vi "2. Simple State Machine Traffic Light.vi"() -> ()   [LabVIEW 2018]
panel:
  in  "stop":bool
  out "Green":bool
  out "Yellow":bool
  out "Red":bool
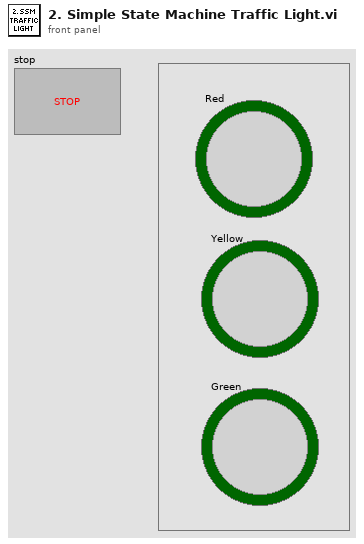
[diagram p1: front panel]
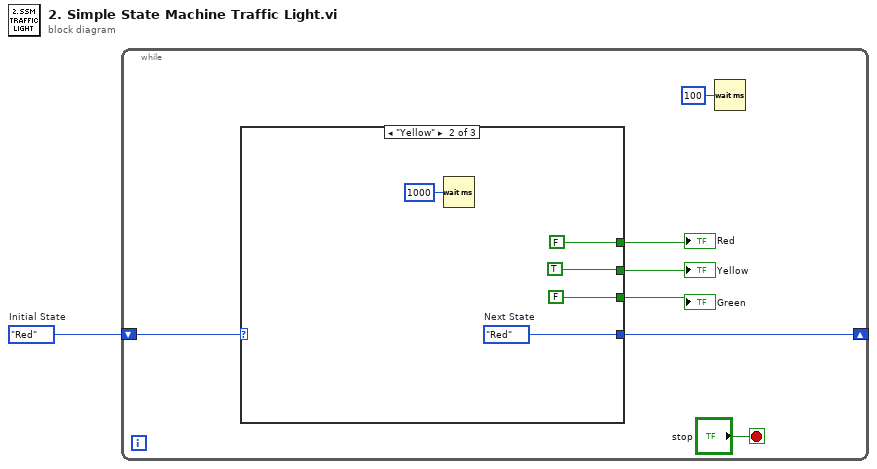
[diagram p0: block diagram]
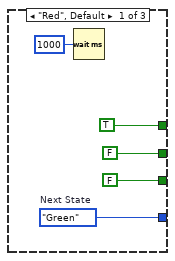
[diagram p2: hidden frame]
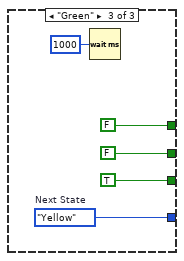
[diagram p3: hidden frame]
diagram:
  w1 = enum16{"Red", "Yellow", "Green"}."Red"  # Initial State
  n1 = while {
    shift-right: [w7] -> _
    shift-left: w1 -> [w8]
    stop <- "stop" stop-if-true
    n2 = case shown="\"Yellow\"" w8 {
      tunnel: [TRUE FALSE FALSE] -> w2
      tunnel: [w12 w17 w22] -> w7
      tunnel: [FALSE TRUE FALSE] -> w4
      tunnel: [FALSE FALSE TRUE] -> w3
      frame "Red", Default {
        w12 = enum16{"Red", "Yellow", "Green"}."Green"  # Next State
        n3 = Wait (ms)(milliseconds to wait=u32 1000) -> ()  [unwired: 1 out]
      }
      frame "Yellow" {
        w17 = enum16{"Red", "Yellow", "Green"}."Red"  # Next State
        n4 = Wait (ms)(milliseconds to wait=u32 1000) -> ()  [unwired: 1 out]
      }
      frame "Green" {
        w22 = enum16{"Red", "Yellow", "Green"}."Yellow"  # Next State
        n5 = Wait (ms)(milliseconds to wait=u32 1000) -> ()  [unwired: 1 out]
      }
    }
    "Red" <- w2
    "Yellow" <- w4
    "Green" <- w3
    n6 = Wait (ms)(milliseconds to wait=u32 100) -> ()  [unwired: 1 out]
  }
